vi "Coord window-Delete coord row.vi"(8 "error in (no error)":errorcluster, 11 "MulticolumnListbox in":refnum<vi>) -> (0 "error out":errorcluster, 3 "MulticolumnListbox out":refnum<vi>)   [LabVIEW 2017]
uses:
  Globals/Coord window-Globals.vi
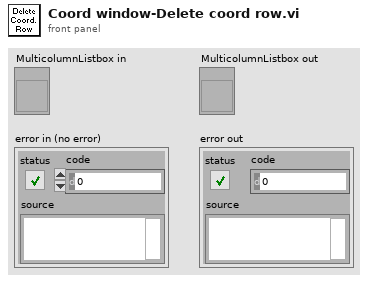
[diagram p1: front panel]
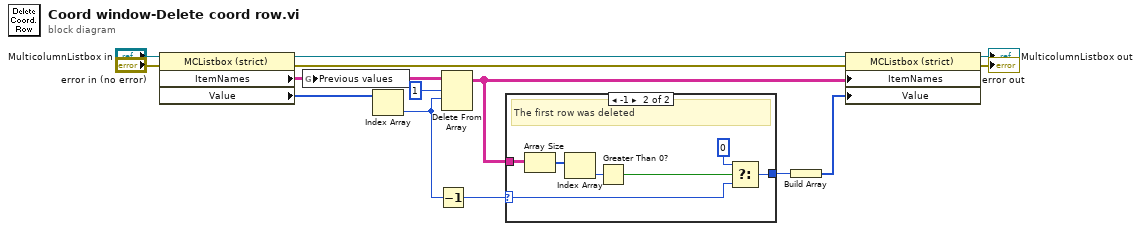
[diagram p0: block diagram]
diagram:
  n1 = property on="Property Node" class="MCListbox (strict)"(reference="MulticolumnListbox in", error in="error in (no error)") -> (reference out=w8:refnum<vi>, error out=w13:errorcluster, "ItemNames"=w1:string[][], "Value"=w6:i32[])
  n2 = global write "Coord window-Globals.vi" "Previous values"(w1) -> ()
  n3 = Index Array(array=w6) -> (element=w9:i32)  [unwired: 1 in]
  n4 = Decrement(x=w9) -> (x-1=w4:i32)
  n5 = Delete From Array(array=w1, length=1, index (row)=w9) -> (array with subset deleted=w2:string[][])  [unwired: 1 in, 1 out]
  n6 = case shown="-1" w4 {
    selector: w4 -> [w15 w18]
    tunnel: [w15 w17] -> w3
    tunnel: w2 -> [_ w22]
    frame Default {
      # "Any row was deleted other than the first one"
    }
    frame -1 {
      # "The first row was deleted"
      n7 = Array Size(array=w22) -> (size(s)=w21:i32[])
      n8 = Index Array(array=w21) -> (element=w20:i32)  [unwired: 1 in]
      n9 = Greater Than 0?(x=w20) -> (x > 0?=w19:bool)
      n10 = Select(t=0, s=w19, f=w18) -> (s? t:f=w17:i32)
    }
  }
  n11 = Build Array(w3) -> (w10:i32[])
  n12 = property on="Property Node" class="MCListbox (strict)"(reference=w8, error in=w13, "ItemNames"=w2, "Value"=w10) -> (reference out=→"MulticolumnListbox out":refnum<vi>, error out=→"error out":errorcluster)
